vi "Sync dynamic editors with array.vi"(9 "Row index":i32, 10 "Array control":refnum<vi>, 11 "Controls":refnum<vi>[](array[refnum])) -> ()   [LabVIEW 2014, in "COSYLib.lvlib"]
doc: "Changes the Y position of a set of front-panel controls to match a row in an Array control.\nIf the selected row number is -1, the controls are hidden."
uses:
  COSYLib.lvlib
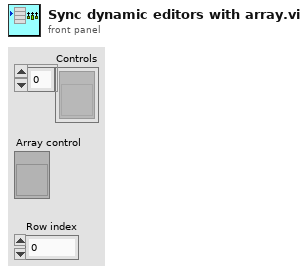
[diagram p1: front panel]
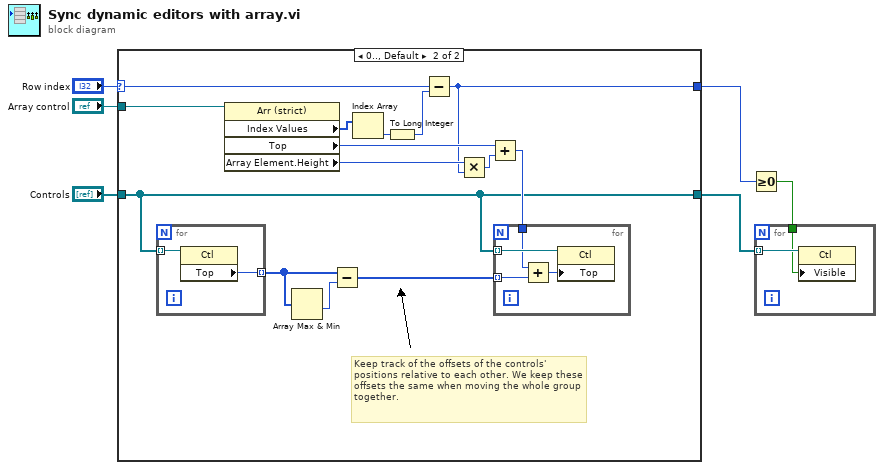
[diagram p0: block diagram]
diagram:
  n1 = case shown="0.., Default" "Row index" {
    selector: "Row index" -> [w8 w11]
    tunnel: "Controls" -> [w7 w14]
    tunnel: "Array control" -> [_ w20]
    tunnel: [w7 w14] -> w3
    tunnel: [w8 w10] -> w2
    frame -1 {
    }
    frame 0.., Default {
      # "Keep track of the offsets of the controls' positions relative to each other. We keep these offsets the same when moving the whole group together."
      n2 = for {
        tunnel: w14 -> [w28] mode=indexing
        tunnel: [w27] -> w22 mode=indexing
        n3 = property class="Ctl"(reference=w28) -> ("Top"=w27:i32)  [unwired: 1 in, 2 out]
      }
      n4 = property class="Arr (strict)"(reference=w20) -> ("Index Values"=w13:u32[], "Top"=w19:i32, "Array Element.Height"=w18:u32)  [unwired: 1 in, 2 out]
      n5 = Array Max & Min(array=w22) -> (min value=w21:i32)  [unwired: 3 out]
      n6 = Subtract(x=w22, y=w21) -> (x-y=w16:i32[])
      n7 = Index Array(array=w13) -> (element=w12:u32)  [unwired: 1 in]
      n8 = To Long Integer(number=w12) -> (32bit integer=w9:i32)
      n9 = Subtract(x=w11, y=w9) -> (x-y=w10:i32)
      n10 = Multiply(x=w18, y=w10) -> (x*y=w17:u32)
      n11 = Add(x=w19, y=w17) -> (x+y=w15:u32)
      n12 = for {
        tunnel: w14 -> [w26] mode=indexing
        tunnel: w16 -> [w25] mode=indexing
        tunnel: w15 -> [w23]
        n13 = Add(x=w23, y=w25) -> (x+y=w24:u32)
        n14 = property class="Ctl"(reference=w26, "Top"=w24) -> ()  [unwired: 1 in, 2 out]
      }
    }
  }
  n15 = Greater Or Equal To 0?(x=w2) -> (x >= 0?=w1:bool)
  n16 = for {
    tunnel: w3 -> [w30] mode=indexing
    tunnel: w1 -> [w29]
    n17 = property class="Ctl"(reference=w30, "Visible"=w29) -> ()  [unwired: 1 in, 2 out]
  }
